vi "Global Log To String(Source Time).vi"(6 "Format String":string="%<%H:%M:%S%3u>T", 10 "Log":T1) -> (3 "Log String":string)   [LabVIEW 2017, in "Communicable State Machine.lvlib"]
uses:
  Communicable State Machine.lvlib
  _Support/Typedef/_CSM_GlobalLog_MSG.ctl
  _Support/Typedef/_CSM_Response Source Message.ctl
  _Support/Typedef/_CSM_GlobalLog_MSG_TYPE.ctl
  _Shared/CSM Shared.lvlib
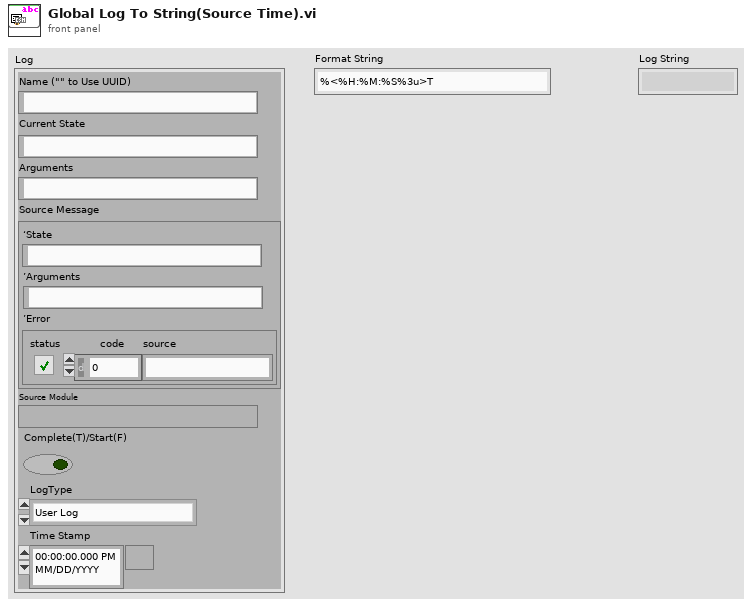
[diagram p1: front panel]
types:
  T1 = typedef "Communicable State Machine.lvlib/_CSM_GlobalLog_MSG.ctl" = cluster{"Name (\"\" to Use UUID)":string, "Current State":string, "Arguments":string, "Source Message":T2, "Source Module":string, "Complete(T)/Start(F)":bool, "LogType":T3, "Time Stamp":timestamp}
  T2 = typedef "Communicable State Machine.lvlib/_CSM_Response Source Message.ctl" = cluster{"‘State":string, "’Arguments":string, "’Error":errorcluster}
  T3 = typedef "Communicable State Machine.lvlib/_CSM_GlobalLog_MSG_TYPE.ctl" = enum16{"User Log", "State Change", "Status", "Interrupt", "Register", "Unregister", "Error Log", "Module Created", "Module Destroyed"}
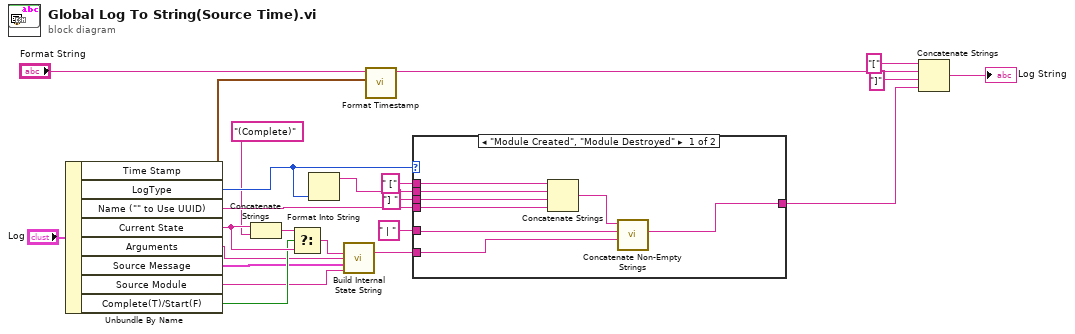
[diagram p0: block diagram]
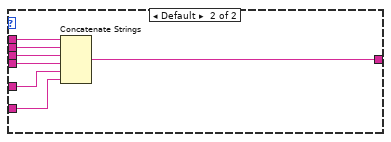
[diagram p2: hidden frame]
diagram:
  n1 = Unbundle By Name("Log") -> ("Time Stamp"=w8:timestamp, "LogType"=w11:T3, "Name (\"\" to Use UUID)"=w13:string, "Current State"=w20:string, "Arguments"=w14:string, "Source Message"=w15:T2, "Source Module"=w16:string, "Complete(T)/Start(F)"=w18:bool)
  n2 = Concatenate Strings(w20, "(Complete)" ("string")) -> (w19:string)
  n3 = Select(t=w19, s=w18, f=w20) -> (s? t:f=w21:string)
  n4 = Format Into String(w11) -> (resulting string=w10:string)  [unwired: 3 in, 1 out]
  n5 = call "Build Internal State String.vi"("State"=w21, "Arguments (\"\")"=w14, "Additional Information"=w15, "Source (\"\")"=w16) -> ("State With Arguments"=w17:string)  [unwired: 11 in]
  n6 = call "Format Timestamp.vi"("Timestamp"=w8, "Format String"="Format String") -> ("String"=w2:string)  [unwired: 9 in]
  n7 = case shown="\"Module Created\", \"Module Destroyed\"" w11 {
    tunnel: w10 -> [w30 w38]
    tunnel: "] " ("string") -> [w29 w37]
    tunnel: " [" ("string") -> [w31 w36]
    tunnel: w13 -> [w28 w35]
    tunnel: [w24 w32] -> w4
    tunnel: w17 -> [w26 w33]
    tunnel: " | " ("string") -> [w25 w34]
    frame "Module Created", "Module Destroyed" {
      n8 = Concatenate Strings(w31, w30, w29, w28) -> (w27:string)
      n9 = call "Concatenate Non-Empty Strings.vi"("String2"=w26, "Seperator(Carriage Return)"=w25, "String1"=w27) -> ("Result String"=w24:string)  [unwired: 5 in]
    }
    frame Default {
      n10 = Concatenate Strings(w36, w38, w37, w35, w34, w33) -> (w32:string)
    }
  }
  n11 = Concatenate Strings("[" ("string"), w2, "]" ("string"), w4) -> (→"Log String":string)
